vi "XY Graph Get Plot Range.vi"(11 "Plot in":cluster{"X Array":dbl[], "Y Array":dbl[]}) -> (3 "Plot Range":T1)   [LabVIEW 2021, in "XY Graph Add-Ons.lvlib"]
uses:
  XY Graph Add-Ons.lvlib
  Plot Range.ctl
  Graphs.lvlib
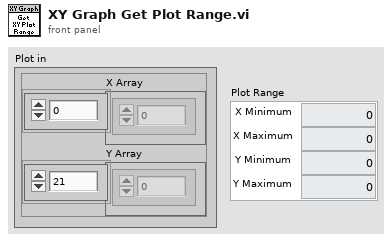
[diagram p1: front panel]
types:
  T1 = typedef "Graphs.lvlib/Plot Range.ctl" = cluster{"X Minimum":dbl, "X Maximum":dbl, "Y Minimum":dbl, "Y Maximum":dbl}
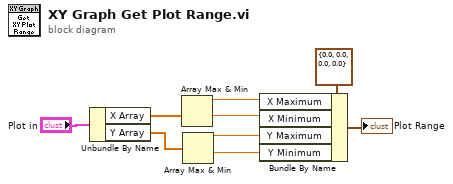
[diagram p0: block diagram]
diagram:
  n1 = Unbundle By Name("Plot in") -> ("X Array"=w2:dbl[], "Y Array"=w1:dbl[])
  n2 = Array Max & Min(array=w2) -> (max value=w6:dbl, min value=w7:dbl)  [unwired: 2 out]
  n3 = Array Max & Min(array=w1) -> (max value=w8:dbl, min value=w9:dbl)  [unwired: 2 out]
  n4 = Bundle By Name(cluster=T1 {"X Minimum"=0.0, "X Maximum"=0.0, "Y Minimum"=0.0, "Y Maximum"=0.0} ("Plot Range"), "X Maximum"=w6, "X Minimum"=w7, "Y Maximum"=w8, "Y Minimum"=w9) -> (→"Plot Range":T1)
